vi "Read from Hardware.vi"(8 "error in (no error)":errorcluster, 10 "Values in":dbl[](array[numeric]), 11 "Ballard ARINC-429 Rx Execution Unit in":refnum<class "Ballard ARINC-429 Rx Execution Unit.lvclass">) -> (0 "error out":errorcluster, 2 "Values out":dbl[](array[numeric]), 3 "Ballard ARINC-429 Rx Execution Unit out":refnum<class "Ballard ARINC-429 Rx Execution Unit.lvclass">)   [LabVIEW 2020, in "Communication Bus Template Engine.lvlib" / "Implementation.lvlib" / "Ballard ARINC-429 Rx Execution Unit.lvclass"]
uses:
  Ballard ARINC-429 Rx Execution Unit.lvclass
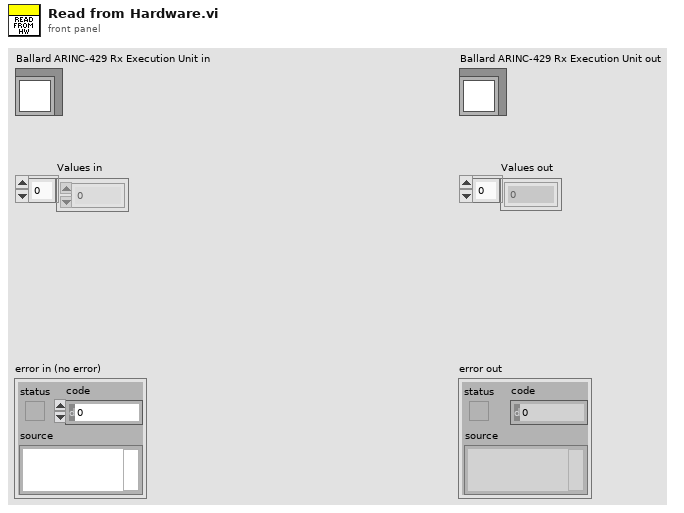
[diagram p1: front panel]
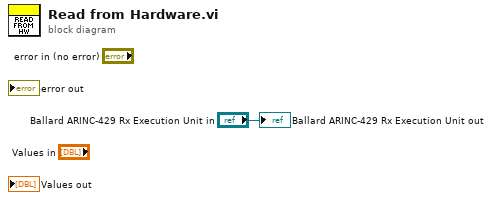
[diagram p0: block diagram]
diagram:
  "Ballard ARINC-429 Rx Execution Unit out" <- "Ballard ARINC-429 Rx Execution Unit in"
